vi "logEventAirStatus.vi"(8 "error in (no error)":errorcluster, 10 "EventAirStatus":T1, 11 "Communicator in":refnum<class "Communicator.lvclass">) -> (0 "error out":errorcluster, 3 "Communicator out":refnum<class "Communicator.lvclass">)   [LabVIEW 2016, in "M1M3SupportCommunicator.lvlib" / "Communicator.lvclass"]
uses:
  Communicator.lvclass
  DataTypes/Topics/EventAirStatus.ctl
  DataTypes/Topics/Parts/Timestamp.ctl
  DataTypes/Topics/M1M3SupportTopics.lvlib
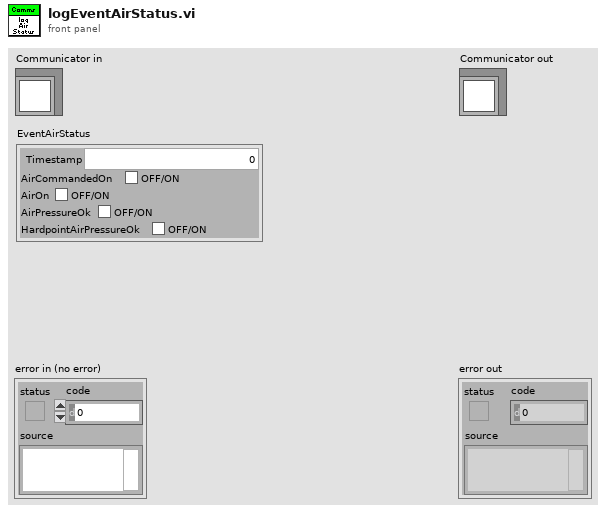
[diagram p1: front panel]
types:
  T1 = typedef "M1M3SupportTopics.lvlib/EventAirStatus.ctl" = cluster{"Timestamp":T2, "AirCommandedOn":bool, "AirOn":bool, "AirPressureOk":bool, "HardpointAirPressureOk":bool}
  T2 = typedef "M1M3SupportTopics.lvlib/Timestamp.ctl" = dbl
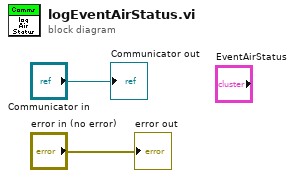
[diagram p0: block diagram]
diagram:
  "error out" <- "error in (no error)"
  "Communicator out" <- "Communicator in"
